vi "toggleSlideState.vi"(8 "error in (no error)":errorcluster {"code" format="Error %.0f"}, 9 "displayListToggleRef":refnum<vi>, 10 "displayListRef":refnum<vi>, 11 "paneRef":refnum<vi>) -> (0 "error out":errorcluster {"code" format="Error %.0f"})   [LabVIEW 2017]
doc: "This VI toggles the slide state of a sliding object. if current state is open, the setSlideState action input = close and the object will slide close and vice versa."
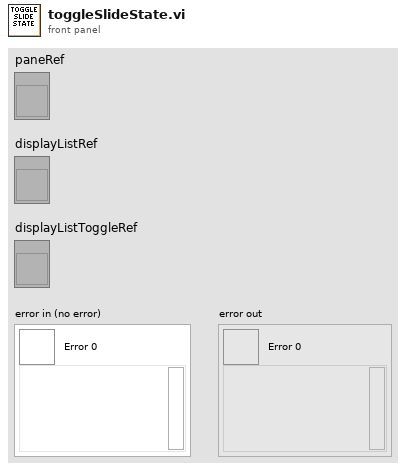
[diagram p1: front panel]
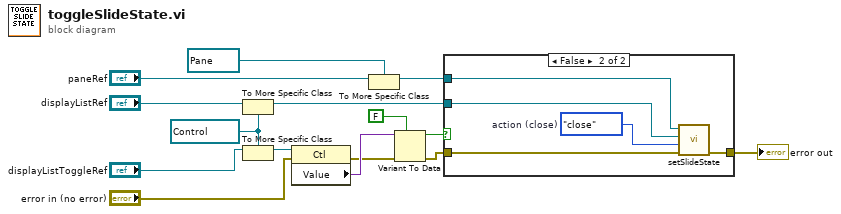
[diagram p0: block diagram]
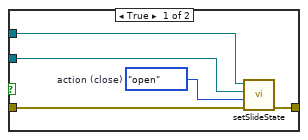
[diagram p2: hidden frame]
diagram:
  w3 = refnum<vi> refnum ("Ctl Refnum")
  n1 = To More Specific Class(target class=w3, reference="displayListRef") -> (specific class reference=w4:refnum<vi>)  [unwired: 1 in, 1 out]
  n2 = To More Specific Class(target class=w3, reference="displayListToggleRef") -> (specific class reference=w1:refnum<vi>)  [unwired: 1 in, 1 out]
  n3 = property class="Ctl"(reference=w1, error in="error in (no error)") -> (error out=w13:errorcluster, "Value"=w15:variant)  [unwired: 1 out]
  n4 = To More Specific Class(target class=refnum<vi> refnum ("Pane Refnum"), reference="paneRef") -> (specific class reference=w6:refnum<vi>)  [unwired: 1 in, 1 out]
  n5 = Variant To Data(error in=w13, type=FALSE, Variant=w15) -> (data=w9:bool, error out=w12:errorcluster)
  n6 = case shown="False" w9 {
    tunnel: w6 -> [w20 w25]
    tunnel: w4 -> [w19 w24]
    tunnel: w12 -> [w18 w23]
    tunnel: [w17 w22] -> w11
    frame True {
      w16 = enum16{"open", "close"}."open"  # action (close)
      n7 = call "setSlideState.vi"("error in (no error)"=w18, "action (close)"=w16, "controlRef"=w19, "paneRef"=w20) -> ("error out"=w17:errorcluster)  [unwired: 6 in, 1 out]
    }
    frame False {
      w21 = enum16{"open", "close"}."close"  # action (close)
      n8 = call "setSlideState.vi"("error in (no error)"=w23, "action (close)"=w21, "controlRef"=w24, "paneRef"=w25) -> ("error out"=w22:errorcluster)  [unwired: 6 in, 1 out]
    }
  }
  "error out" <- w11
